vi "UDP Factory.vi"(8 "error in (no error)":errorcluster, 10 "UDP settings":T1) -> (0 "error out":errorcluster, 3 "protocol out":refnum<class "Protocol Parent.lvclass">)   [LabVIEW 2018, in "Protocols.lvlib" / "UDP.lvclass"]
doc: "Instantiates a new UPD Protocol object using the provided UDP settings."
uses:
  UDP.lvclass
  UDP Settings.ctl
  Protocol Parent/Protocol Parent.lvclass
  D:/GitRepository/niveristand-instrument-addon-classes/Source/Protocols/Protocol Parent/Protocol Parent.lvclass
  UDP.lvclass/UDP.ctl
  Data Access/Write Local IP Address.vi
  Data Access/Write Local Port.vi
  Data Access/Write Target IP Address.vi
  Data Access/Write Target Port.vi
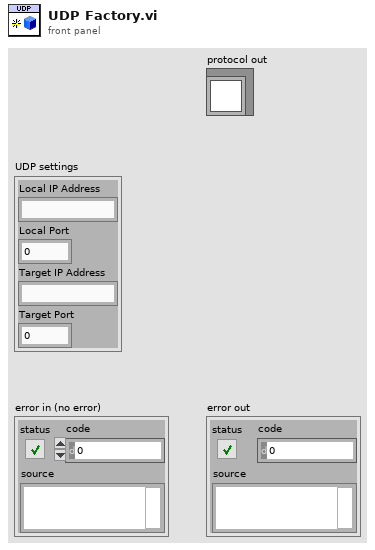
[diagram p1: front panel]
types:
  T1 = typedef "Protocols.lvlib/UDP.lvclass/UDP Settings.ctl" = cluster{"Local IP Address":string, "Local Port":u16, "Target IP Address":string, "Target Port":u16}
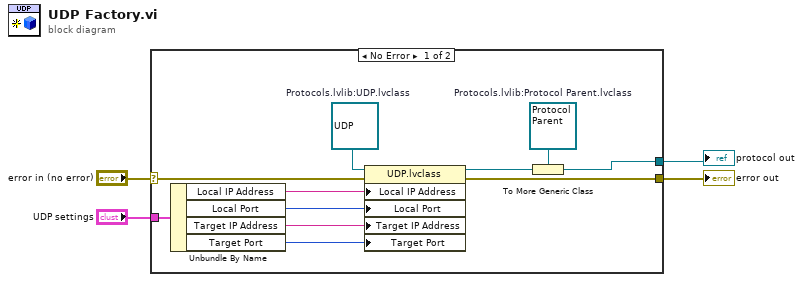
[diagram p0: block diagram]
diagram:
  n1 = case shown="No Error" "error in (no error)" {
    selector: "error in (no error)" -> [w9 w16]
    tunnel: "UDP settings" -> [w15 _]
    tunnel: [w7 w16] -> w3
    tunnel: [w5 _] -> w1
    frame No Error {
      w6 = refnum<class "Protocol Parent.lvclass"> refnum  # Protocols.lvlib:Protocol Parent.lvclass
      w14 = refnum<class "UDP.lvclass"> refnum  # Protocols.lvlib:UDP.lvclass
      n2 = Unbundle By Name(w15) -> ("Local IP Address"=w10:string, "Local Port"=w11:u16, "Target IP Address"=w12:string, "Target Port"=w13:u16)
      n3 = property class="UDP.lvclass"(reference=w14, error in=w9, "Local IP Address"=w10, "Local Port"=w11, "Target IP Address"=w12, "Target Port"=w13) -> (reference out=w8:refnum<class "UDP.lvclass">, error out=w7:errorcluster)
      n4 = To More Generic Class(target class=w6, reference=w8) -> (generic class reference=w5:refnum<class "Protocol Parent.lvclass">)
    }
    frame Error {
    }
  }
  "error out" <- w3
  "protocol out" <- w1
